vi "PLC.ChangeOver.vi"(7 "Idx":i32, 8 "error in":errorcluster, 10 "Slot":i32, 11 "Data_in":T1={"Status"={"Idx"=0, "ConnRef"=0, "State"=enum."Off", "LiveBitTimer"=timestamp(0 s since 1904-01-01)}, "Sets"={"Enable"=FALSE, "IP"="", "Rack"=0, "Slot"=0, "LifeBitTimer_s"=0.0, "DataBlockAddr_PCStatus"=0, "DataBlockAddr_PLCStatus"=1, "DataBlockAddr_PLCNewData"=[], "DataBlockSize_PLCNewData"=[], "DataBlockAddr_PLCChangeOver"=[], "DataBlockSize_PLCChangeOver"=[], "DataBlockAddr_PCChangeOver"=[], "DataBlockAddr_PLCCheckStatus"=[], "DataBlockSize_PLCCheckStatus"=[], "DataBlockAddr_PCCheckStatus"=[], "System"=""}, "PCstatus"={"General"={"LifeBit"=FALSE, "DbRun"=FALSE}, "Stations"=[]}, "PLCstatus"={"General"={"LifeBit"=FALSE}, "Stations"=[]}}) -> (0 "error out":errorcluster, 3 "Data_out":T1={"Status"={"Idx"=0, "ConnRef"=0, "State"=enum."Off", "LiveBitTimer"=timestamp(0 s since 1904-01-01)}, "Sets"={"Enable"=FALSE, "IP"="", "Rack"=0, "Slot"=0, "LifeBitTimer_s"=0.0, "DataBlockAddr_PCStatus"=0, "DataBlockAddr_PLCStatus"=1, "DataBlockAddr_PLCNewData"=[], "DataBlockSize_PLCNewData"=[], "DataBlockAddr_PLCChangeOver"=[], "DataBlockSize_PLCChangeOver"=[], "DataBlockAddr_PCChangeOver"=[], "DataBlockAddr_PLCCheckStatus"=[], "DataBlockSize_PLCCheckStatus"=[], "DataBlockAddr_PCCheckStatus"=[], "System"=""}, "PCstatus"={"General"={"LifeBit"=FALSE, "DbRun"=FALSE}, "Stations"=[]}, "PLCstatus"={"General"={"LifeBit"=FALSE}, "Stations"=[]}})   [LabVIEW 2016]
doc: "Get test results (measurement values) from PLC and save to database\n\nWabco 2017 All right reserved\nAuthor: maciej.szupienko@wabco-auto.com"
uses:
  PLC.Data.ctl
  PLC.Data.Status.ctl
  PLC.State.ctl
  PLC.Data.Sets.ctl
  LowLevel/PLC.DataBlock.PCstatus.ctl
  LowLevel/PLC.DataBlock.PCstatus.General.ctl
  LowLevel/PLC.DataBlock.PCstatus.Station.ctl
  LowLevel/PLC.DataBlock.PLCstatus.ctl
  LowLevel/PLC.DataBlock.PLCstatus.General.ctl
  LowLevel/PLC.DataBlock.PLCstatus.Station.ctl
  LowLevel/PLC.DataBlock.PLCchangeover.ctl
  LowLevel/PLC.DataBlock.PCchangeover.ctl
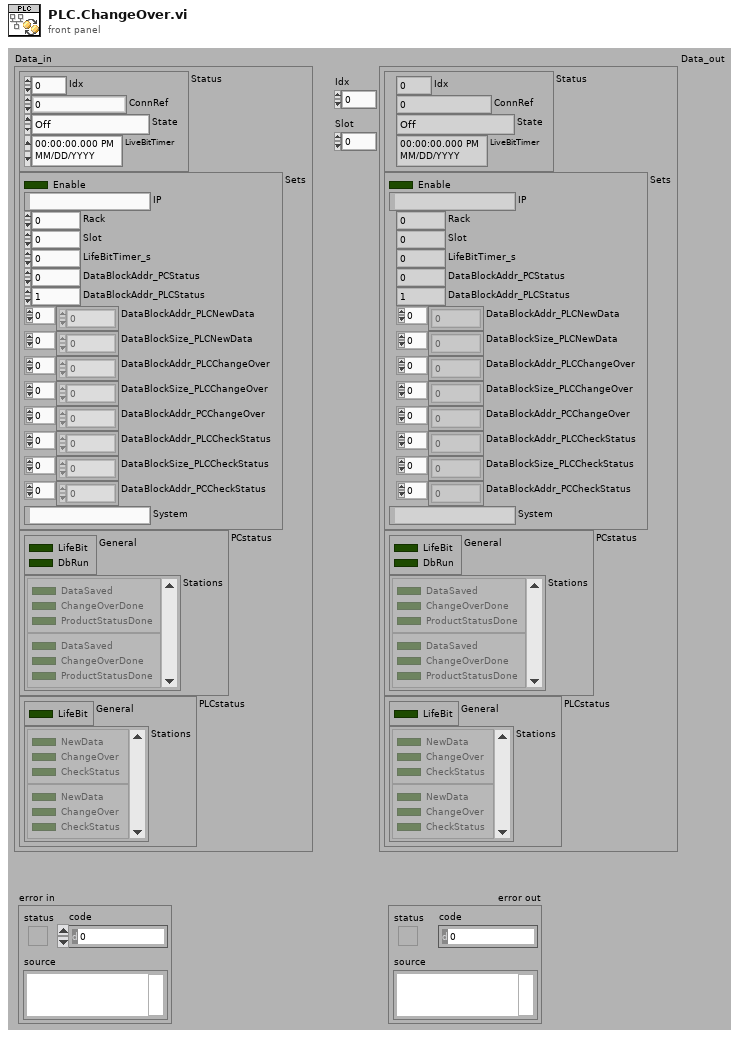
[diagram p1: front panel]
types:
  T1 = typedef "PLC.Data.ctl" = cluster{"Status":T2, "Sets":T4, "PCstatus":T5, "PLCstatus":T8}
  T2 = typedef "PLC.Data.Status.ctl" = cluster{"Idx":i32, "ConnRef":u64, "State":T3, "LiveBitTimer":timestamp}
  T3 = typedef "PLC.State.ctl" = enum32{"Off", "Error", "Idle", "Run"}
  T4 = typedef "PLC.Data.Sets.ctl" = cluster{"Enable":bool, "IP":string, "Rack":i32, "Slot":i32, "LifeBitTimer_s":dbl, "DataBlockAddr_PCStatus":i32, "DataBlockAddr_PLCStatus":i32, "DataBlockAddr_PLCNewData":i32[], "DataBlockSize_PLCNewData":i32[], "DataBlockAddr_PLCChangeOver":i32[], "DataBlockSize_PLCChangeOver":i32[], "DataBlockAddr_PCChangeOver":i32[], "DataBlockAddr_PLCCheckStatus":i32[], "DataBlockSize_PLCCheckStatus":i32[], "DataBlockAddr_PCCheckStatus":i32[], "System":string}
  T5 = typedef "PLC.DataBlock.PCstatus.ctl" = cluster{"General":T6, "Stations":T7[]}
  T6 = typedef "PLC.DataBlock.PCstatus.General.ctl" = cluster{"LifeBit":bool, "DbRun":bool}
  T7 = typedef "PLC.DataBlock.PCstatus.Station.ctl" = cluster{"DataSaved":bool, "ChangeOverDone":bool, "ProductStatusDone":bool}
  T8 = typedef "PLC.DataBlock.PLCstatus.ctl" = cluster{"General":T9, "Stations":T10[]}
  T9 = typedef "PLC.DataBlock.PLCstatus.General.ctl" = cluster{"LifeBit":bool}
  T10 = typedef "PLC.DataBlock.PLCstatus.Station.ctl" = cluster{"NewData":bool, "ChangeOver":bool, "CheckStatus":bool}
  T11 = typedef "PLC.DataBlock.PCchangeover.ctl" = cluster{"TP_Size":u8, "TV_Size":u8, "TP":sgl[], "TVL":sgl[], "TVH":sgl[]}
  T12 = typedef "PLC.DataBlock.PLCchangeover.ctl" = cluster{"Ref":string}
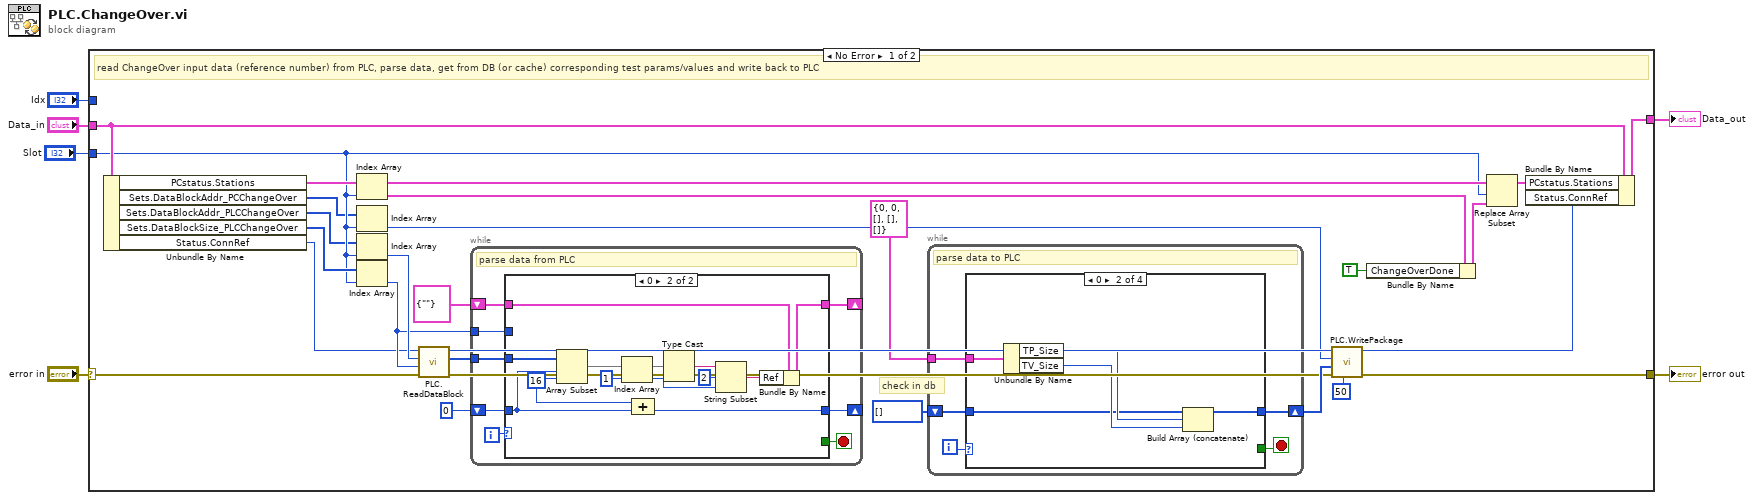
[diagram p0: block diagram]
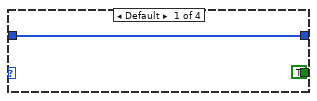
[diagram p2: hidden frame]
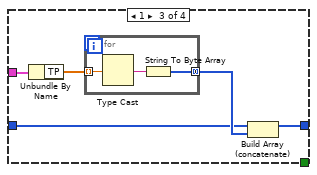
[diagram p3: hidden frame]
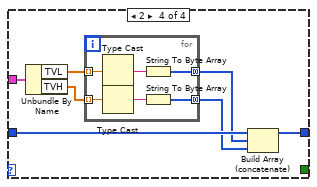
[diagram p4: hidden frame]
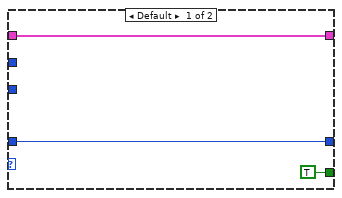
[diagram p5: hidden frame]
diagram:
  n1 = case shown="No Error" "error in" {
    selector: "error in" -> [w32 w91]
    tunnel: [w20 w91] -> w3
    tunnel: "Data_in" -> [w30 w90]
    tunnel: [w33 w90] -> w5
    tunnel: "Idx" -> [_ _]
    tunnel: "Slot" -> [w16 _]
    frame No Error {
      # "check in db"
      # "read ChangeOver input data (reference number) from PLC, parse data, get from DB (or cache) corresponding test params/values and write back to PLC"
      n2 = Unbundle By Name(w30) -> ("PCstatus.Stations"=w17:T7[], "Sets.DataBlockAddr_PCChangeOver"=w13:i32[], "Sets.DataBlockAddr_PLCChangeOver"=w14:i32[], "Sets.DataBlockSize_PLCChangeOver"=w22:i32[], "Status.ConnRef"=w12:u64)
      n3 = Index Array(array=w17, index=w16) -> (element=w28:T7)
      n4 = Index Array(array=w13, index=w16) -> (element=w11:i32)
      n5 = Index Array(array=w14, index=w16) -> (element=w31:i32)
      n6 = Index Array(array=w22, index=w16) -> (element=w23:i32)
      n7 = call "PLC.ReadDataBlock.vi"("error in (no error)"=w32, "Amount (1)"=w23, "Block"=w31, "Ref"=w12) -> ("error out"=w7:errorcluster, "data out"=w26:u8[], "ref out"=w21:u64)  [unwired: 5 in]
      n8 = while {
        tunnel: w26 -> [w69]
        shift-right: [w72] -> _
        shift-left: 0 -> [w73]
        shift-right: [w71] -> _
        shift-left: T12 {"Ref"=""} ("element") -> [w70]
        tunnel: w23 -> [w68]
        i -> [w74]
        stop <- w67 stop-if-true
        # "parse data from PLC"
        n9 = case shown="0" w74 {
          tunnel: w73 -> [w76 w80]
          tunnel: [w76 w79] -> w72
          tunnel: [w77 w89] -> w71
          tunnel: w70 -> [w77 w88]
          tunnel: w69 -> [_ w83]
          tunnel: w68 -> [_ _]
          tunnel: [TRUE _] -> w67
          frame Default {
          }
          frame 0 {
            w81 = 16 ("length")
            n10 = Array Subset(array=w83, index=w80, length=w81) -> (w85:u8[])
            n11 = Index Array(array=w85, index=1) -> (element=w78:u8)
            n12 = Compound Arithmetic op=ADD(w81, w80) -> (w79:i32)
            n13 = Type Cast(x=w85) -> (*(type *) &x=w84:string)  [unwired: 1 in]
            n14 = String Subset(string=w84, offset (0)=2, length (rest)=w78) -> (substring=w82:string)
            n15 = Bundle By Name(cluster=w88, "Ref"=w82) -> (w89:T12)
          }
        }
      }
      n16 = while {
        tunnel: T11 {"TP_Size"=0, "TV_Size"=0, "TP"=[], "TVL"=[], "TVH"=[]} ("PCchangeover") -> [w37]
        shift-right: [w35] -> w10
        shift-left: u8[] [] ("data in") -> [w34]
        i -> [w38]
        stop <- w36 stop-if-true
        # "parse data to PLC"
        n17 = case shown="0" w38 {
          tunnel: w37 -> [_ w45 w50 w60]
          tunnel: [TRUE _ _ _] -> w36
          tunnel: [w39 w42 w46 w57] -> w35
          tunnel: w34 -> [w39 w41 w47 w58]
          frame Default {
          }
          frame 0 {
            n18 = Unbundle By Name(w45) -> ("TP_Size"=w44:u8, "TV_Size"=w43:u8)
            n19 = Build Array (concatenate)(w41, w44, w43) -> (w42:u8[])
          }
          frame 1 {
            n20 = Unbundle By Name(w50) -> ("TP"=w49:sgl[])
            n21 = for {
              tunnel: w49 -> [w53] mode=indexing
              tunnel: [w51] -> w48 mode=concatenating
              n22 = Type Cast(x=w53) -> (*(type *) &x=w52:string)  [unwired: 1 in]
              n23 = String To Byte Array(string=w52) -> (unsigned byte array=w51:u8[])
            }
            n24 = Build Array (concatenate)(w47, w48) -> (w46:u8[])
          }
          frame 2 {
            n25 = Unbundle By Name(w60) -> ("TVL"=w59:sgl[], "TVH"=w56:sgl[])
            n26 = for {
              tunnel: w59 -> [w66] mode=indexing
              tunnel: [w64] -> w54 mode=concatenating
              tunnel: w56 -> [w61] mode=indexing
              tunnel: [w63] -> w55 mode=concatenating
              n27 = Type Cast(x=w66) -> (*(type *) &x=w65:string)  [unwired: 1 in]
              n28 = Type Cast(x=w61) -> (*(type *) &x=w62:string)  [unwired: 1 in]
              n29 = String To Byte Array(string=w65) -> (unsigned byte array=w64:u8[])
              n30 = String To Byte Array(string=w62) -> (unsigned byte array=w63:u8[])
            }
            n31 = Build Array (concatenate)(w58, w54, w55) -> (w57:u8[])
          }
        }
      }
      n32 = call "PLC.WritePackage.vi"("max package size  (0: full)"=50 ("max package size  (0: all)"), "error in (no error)"=w7, "data"=w10, "addr"=w11, "Ref in"=w21) -> ("error out"=w20:errorcluster, "Ref out"=w18:u64)  [unwired: 5 in]
      n33 = Bundle By Name(cluster=w28, "ChangeOverDone"=TRUE) -> (w27:T7)
      n34 = Replace Array Subset(array=w17, new element=w27, index=w16) -> (w29:T7[])
      n35 = Bundle By Name(cluster=w30, "PCstatus.Stations"=w29, "Status.ConnRef"=w18) -> (w33:T1)
    }
    frame Error {
    }
  }
  "error out" <- w3
  "Data_out" <- w5
